vi "PH_O2_Watch.panel.vi"(0 "object ref":refnum<vi>, 5 "error in (no error)":errorcluster) -> (19 "error out":errorcluster)   [LabVIEW 2014, in "PH_O2_Watch.lvlib"]
doc: "By this VI an oxyd measurement device can be monitored. \n\n\n\n\"Delete Instance\" disconnects and removes the instance from the PCS.\n\nThis VI has no machine safety relevant logig: in case of any alarm, for example, nothing is done automatically.\n\nLicense Agreement for this software:\n\nCopyright (C)\nGesellschaft für Schwerionenforschung, GSI\nPlanckstr. 1\n64291 Darmstadt\nGermany\n\nContact: D.Beck@gsi.de \n\nThis program is free software; you can redistribute it and/or modify it under the terms of the GNU General Public License as published by the Free Software Foundation; either version 2 of the license, or (at your option) any later version.\n\nThis program is distributed in the hope that it will be useful, but WITHOUT ANYW ARRANTY; without even the implied warranty of MERCHANTABILITY or FITNESS FOR A PARTICULAR PURPOSE. See the GNU General License for more details (http://www.gnu.org).\n\nGesellschaft für Schwerionenforschung, GSI\nPlanckstr. 1, 64291 Darmstadt, Germany\nFor all questions and ideas contact: M.Richter@gsi.de, H.Brand@gsi.de or D.Beck@gsi.de.\nLast update: 18-DEC-2002"
uses:
  PH_O2_Watch.lvlib
  PH_Basics/PH_StatusHandler/PH_StatusHandler.GUI element.ctl
  CS_Core/CSObj/CSObj.lvlib
  PH_Basics/PH_Common/PH_Common.lvlib
  PH_Basics/PH_Class/PH_Class.lvlib
  PH_Basics/PH_PSDBWriter/PH_PSDBWriter.lvlib
  PH_Basics/PH_StatusHandler/PH_StatusHandler.lvlib
panel:
  out "PSDB Status":u32(colorbox) caption="PSDB"
  out "Limit":dbl format="%#_3g"
  out "Concentration":dbl format="%#_3g"
  out "Status":T1 caption="Enabling State"
  in  "Exit":bool
  out "Failure":u32(colorbox)=6618880
  in  "Delete":bool
  out "Alert":u32(colorbox)=6618880
  out "PreAlert":u32(colorbox)=6618880
  # "PCS"
  # "3.40"
  # "%"
  # "%"
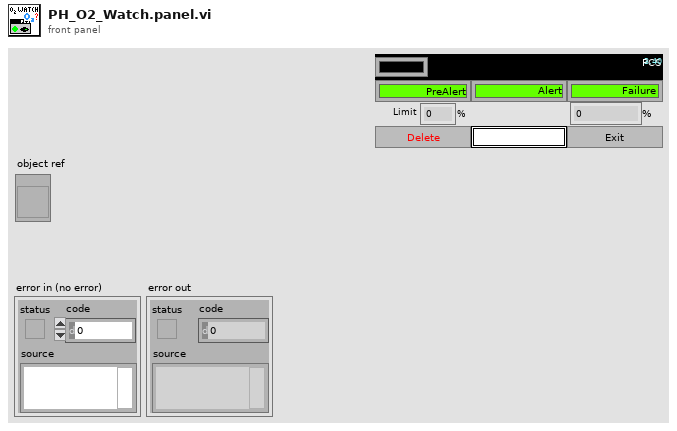
[diagram p1: front panel]
types:
  T1 = typedef "PH_StatusHandler.lvlib/PH_StatusHandler.GUI element.ctl" = u16
  T2 = typedef "PH_O2_Watch.lvlib/PH_O2_Watch.i attribute.ctl" = cluster{"GUI Refs":cluster{"PreAlert":refnum<vi>, "Alert":refnum<vi>, "Failure":refnum<vi>, "Concentration":refnum<vi>, "Delete":refnum<vi>, "Limit":refnum<vi>}, "State PreAlert":T3, "State Alert":T3, "State Failure":T3, "Concentration":dbl, "Limit":dbl}
  T3 = typedef "PH_StatusHandler.lvlib/PH_StatusHandler.Status.ctl" = i16
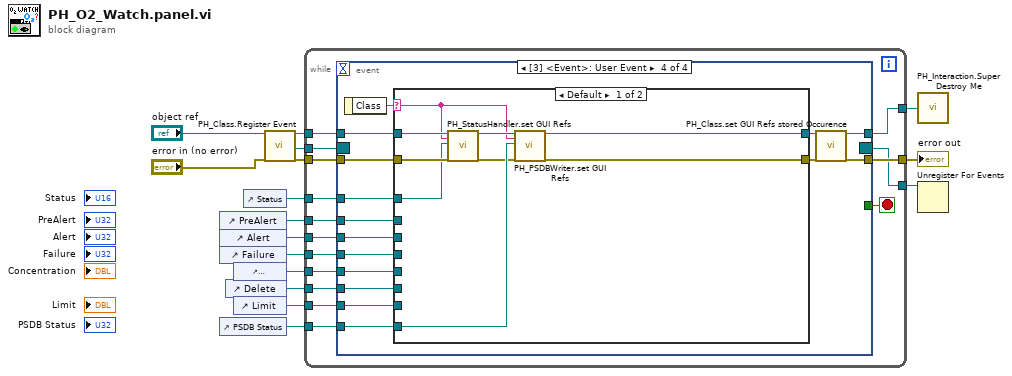
[diagram p0: block diagram]
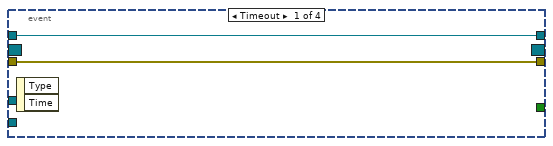
[diagram p2: hidden frame]
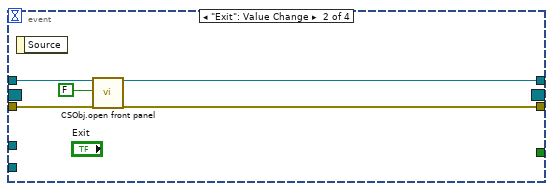
[diagram p3: hidden frame]
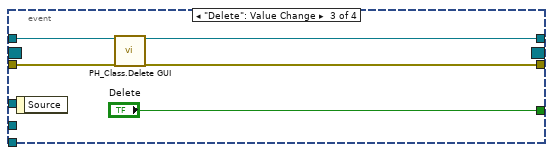
[diagram p4: hidden frame]
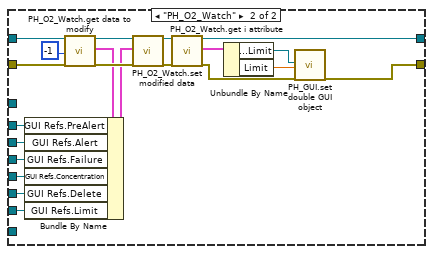
[diagram p5: hidden frame]
diagram:
  n1 = control-ref of="PreAlert"() -> (w10:refnum<vi>)
  n2 = control-ref of="Alert"() -> (w9:refnum<vi>)
  n3 = control-ref of="Failure"() -> (w8:refnum<vi>)
  n4 = control-ref of="PSDB Status"() -> (w4:refnum<vi>)
  n5 = control-ref of="Delete"() -> (w6:refnum<vi>)
  n6 = control-ref of="Concentration"() -> (w7:refnum<vi>)
  n7 = control-ref of="Limit"() -> (w5:refnum<vi>)
  n8 = control-ref of="Status"() -> (w1:refnum<vi>)
  n9 = call "PH_Class.Register Event.vi"("i ref in"="object ref", "error in (no error)"="error in (no error)") -> ("i ref out"=w14:refnum<vi>, "Event Registration Refnum"=w12:refnum<event-registration>, "error out"=w13:errorcluster)  [unwired: 15 in]
  n10 = while {
    tunnel: w14 -> [w28]
    tunnel: [w27] -> w16
    tunnel: w13 -> [w30]
    tunnel: [w29] -> w15
    tunnel: w12 -> [w26]
    tunnel: [w25] -> w11
    tunnel: w10 -> [w24]
    tunnel: w9 -> [w23]
    tunnel: w8 -> [w22]
    tunnel: w7 -> [w21]
    tunnel: w6 -> [w20]
    tunnel: w1 -> [w19]
    tunnel: w5 -> [w18]
    tunnel: w4 -> [w17]
    stop <- w31 stop-if-true
    n11 = event shown="[3] <Event>: User Event" {
      selector: w26 -> [_ _ _ _]
      dyn-events: [_ _ _ _] -> w25
      timeout: _ -> [_ _ _ _]
      tunnel: [_ _ "Delete" _] -> w31
      tunnel: w28 -> [w32 w37 w42 w58]
      tunnel: w30 -> [w33 w36 w41 w57]
      tunnel: [w33 w35 w40 w46] -> w29
      tunnel: [w32 w34 w39 w47] -> w27
      tunnel: w24 -> [_ _ _ w56]
      tunnel: w23 -> [_ _ _ w55]
      tunnel: w22 -> [_ _ _ w54]
      tunnel: w21 -> [_ _ _ w53]
      tunnel: w20 -> [_ _ _ w52]
      tunnel: w19 -> [_ _ _ w51]
      tunnel: w18 -> [_ _ _ w50]
      tunnel: w17 -> [_ _ _ w44]
      event Timeout {
        n12 = event-data() -> ()  [unwired: 1 in, 2 out]
      }
      event "Exit": Value Change {
        n13 = event-data() -> ()  [unwired: 1 in, 1 out]
        n14 = call "CSObj.open front panel.vi"("i ref in"=w37, "frontPanelOpen"=FALSE ("front panel open"), "error in (no error)"=w36) -> ("i ref out"=w34:refnum<vi>, "error out"=w35:errorcluster)  [unwired: 15 in]
      }
      event "Delete": Value Change {
        n15 = event-data() -> ()  [unwired: 1 in, 1 out]
        n16 = call "PH_Class.Delete GUI.vi"("VI in"=w42, "error in (no error)"=w41) -> ("VI out"=w39:refnum<vi>, "error out"=w40:errorcluster)  [unwired: 16 in]
      }
      event User Event {
        n17 = event-data() -> ("Class"=w45:string)  [unwired: 1 in]
        n18 = case shown="Default" w45 {
          selector: w45 -> [w60 _]
          tunnel: w58 -> [w62 w83]
          tunnel: w57 -> [w67 w82]
          tunnel: w56 -> [_ w81]
          tunnel: w55 -> [_ w80]
          tunnel: w54 -> [_ w79]
          tunnel: w53 -> [_ w78]
          tunnel: w52 -> [_ w77]
          tunnel: w51 -> [w59 _]
          tunnel: w50 -> [_ w76]
          tunnel: [w65 w68] -> w49
          tunnel: [w66 w69] -> w48
          tunnel: w44 -> [w64 _]
          frame Default {
            n19 = call "PH_StatusHandler.set GUI Refs.vi"("i ref in"=w62, "Class"=w60, "GUI Ref"=w59, "error in (no error)"=w67) -> ("i ref out"=w61:refnum<vi>, "error out"=w63:errorcluster)  [unwired: 14 in]
            n20 = call "PH_PSDBWriter.set GUI Refs.vi"("i ref in"=w61, "Class"=w60, "Ref PSDB Status"=w64, "error in"=w63) -> ("i ref out"=w66:refnum<vi>, "error out"=w65:errorcluster)  [unwired: 14 in]
          }
          frame "PH_O2_Watch" {
            n21 = call "PH_O2_Watch.get data to modify.vi"("i ref in"=w83, "ms timeout (10000)"=-1, "error in (no error)"=w82) -> ("i ref out"=w88:refnum<vi>, "i attribute"=w86:T2, "error out"=w87:errorcluster)  [unwired: 13 in, 1 out]
            n22 = Bundle By Name(cluster=w86, "GUI Refs.PreAlert"=w81, "GUI Refs.Alert"=w80, "GUI Refs.Failure"=w79, "GUI Refs.Concentration"=w78, "GUI Refs.Delete"=w77, "GUI Refs.Limit"=w76) -> (w85:T2)
            n23 = call "PH_O2_Watch.set modified data.vi"("i ref in"=w88, "i attribute"=w85, "error in (no error)"=w87) -> ("i ref out"=w70:refnum<vi>, "error out"=w71:errorcluster)  [unwired: 15 in]
            n24 = call "PH_O2_Watch.get i attribute.vi"("i ref in"=w70, "error in (no error)"=w71) -> ("i ref out"=w69:refnum<vi>, "i attribute"=w72:T2, "error out"=w73:errorcluster)  [unwired: 15 in]
            n25 = Unbundle By Name(w72) -> ("GUI Refs.Limit"=w74:refnum<vi>, "Limit"=w75:dbl)
            n26 = call "PH_GUI.set double GUI object.vi"("GUI object Ref"=w74, "value"=w75, "error in (no error)"=w73) -> ("error out"=w68:errorcluster)  [unwired: 16 in]
          }
        }
        n27 = call "PH_Class.set GUI Refs stored Occurence.vi"("i ref in"=w48, "error in (no error)"=w49) -> ("i ref out"=w47:refnum<vi>, "error out"=w46:errorcluster)  [unwired: 16 in]
      }
    }
  }
  "error out" <- w15
  n28 = call "PH_Interaction.Super Destroy Me.vi"("i ref out"=w16) -> ()
  n29 = Unregister For Events(event registration refnum=w11) -> ()  [unwired: 1 in, 1 out]
